vi "VPA QC Flow Calibration.vi"(9 "DAQ Ref Cluster":T2, 10 "State In":T4) -> (2 "State Out":T4)   [LabVIEW 2013]
uses:
  Controls/VPA QC State Data Cluster.ctl
  Controls/VPA QC General Cluster.ctl
  Controls/VPA QC State Enum.ctl
  Controls/VPA QC Bool Cluster.ctl
  Controls/VPA QC DAQ Ref Cluster.ctl
  Controls/VPA QC Scale Communication Settings DVR.ctl
  Controls/VPA QC Scale Communication Settings.ctl
  Controls/VPA QC Flow Rate Data Cluster.ctl
  Controls/VPA QC Volume Timer Enum.ctl
panel:
  in  "Flow Data Array":T1[](array[typedef])
  in  "Set 4":bool
  in  "Set 3":bool
  in  "Set 2":bool
  in  "Set 1":bool
  in  "Density of Fluid":dbl=0.996
  out "Cust 2 Elapsed Time":dbl format="%<%M:%S%1u>t"
  in  "Cust Rate 2":dbl=0.01 caption="ML/Min"
  in  "Cust Rate 1":dbl=0.1 caption="ML/Min"
  out "% Dif 4":dbl
  out "Volume 4":dbl caption="Flow Rate (mL/min)" format="%5.2g"
  out "Running 4":bool
  in  "Cust Ready 2":bool caption="Custom Timer2"
  out "Rate 4":dbl
  in  "Flow Rate 4":dbl caption="Flow Rate (mL/min)"
  out "Calc Vol 4":dbl
  out "% Difference Cust1":dbl
  out "Volume 3":dbl caption="Flow Rate (mL/min)" format="%5.2g"
  out "Running 3":bool
  in  "Cust Ready 1":bool caption="Custom Timer1"
  out "Cust 1 Calculated \nFlow Rate (mL/min)":dbl
  out "Cust 1 Elapsed Time":dbl format="%<%M:%S%1u>t"
  in  "Flow Rate 3":dbl caption="Flow Rate (mL/min)"
  out "Vol 3":dbl
  out "A Side Calibration Constant":dbl caption="Flow Rate (mL/min)"
  out "B Side Calibration Constant":dbl caption="Flow Rate (mL/min)"
  out "% Difference 100":dbl
  out "% Difference 50":dbl caption="% Difference"
  out "Volume 2":dbl caption="Flow Rate (mL/min)" format="%5.2g"
  out "Reported\nVolume":dbl caption="Flow Rate (mL/min)" format="%5.2g"
  in  "Cancel":bool
  in  "Save":bool
  out "Running 2":bool
  out "Running":bool
  in  "Ready 100%":bool caption="95% Flow Rate"
  in  "Ready 50%":bool caption="50% Flow Rate"
  out "Calculated Flow Rate\n(mL/min) 2":dbl
  out "Calculated Flow\n Rate (mL/min)":dbl
  out "Elapsed Time 2":dbl format="%<%M:%S%1u>t"
  out "Elapsed Time":dbl format="%<%M:%S%1u>t"
  in  "Flow Rate 2":dbl caption="Flow Rate (mL/min)"
  in  "Flow Rate\n(mL/min)":dbl caption="Flow Rate (mL/min)"
  out "Vol 2":dbl
  out "Vol 1":dbl caption="Measured\nVolume\n(mass/density)"
  # "Flow Rate Test"
  # "1. Go to Constant Flow Mode and flow to some volume at 50%  max flow, 95% max flow, and two low flow rates. Calculate the flow rate from the measured volume and time."
  # "Enter Pump\nReported Values"
  # "Calculated Values"
  # "Assembly Checklist"
  # "Assembly Checklist"
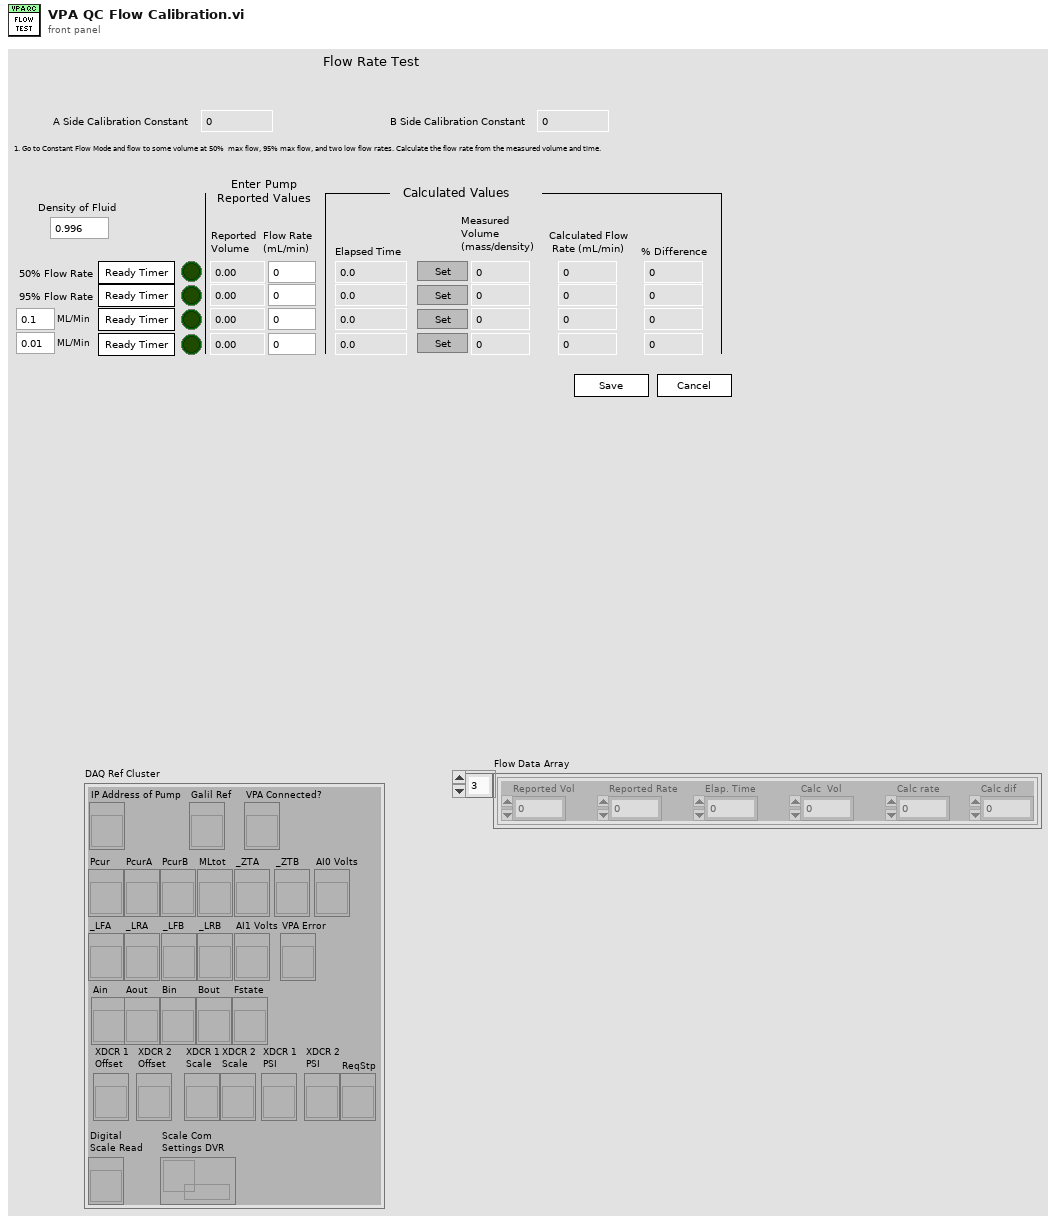
[diagram p1: front panel]
types:
  T1 = typedef "VPA QC Flow Rate Data Cluster.ctl" = cluster{"Reported Vol":dbl, "Reported Rate":dbl, "Elap. Time":dbl, "Calc  Vol":dbl, "Calc rate":dbl, "Calc dif":dbl}
  T2 = typedef "VPA QC DAQ Ref Cluster.ctl" = cluster{"IP Address of Pump":refnum<vi>, "Galil Ref":refnum<vi>, "VPA Connected?":refnum<vi>, "Pcur":refnum<vi>, "PcurA":refnum<vi>, "PcurB":refnum<vi>, "MLtot":refnum<vi>, "_LFA":refnum<vi>, "_LRA":refnum<vi>, "_LFB":refnum<vi>, "_LRB":refnum<vi>, "_ZTA":refnum<vi>, "_ZTB":refnum<vi>, "AI0 Volts":refnum<vi>, "AI1 Volts":refnum<vi>, "VPA Error":refnum<vi>, "Ain":refnum<vi>, "Aout":refnum<vi>, "Bin":refnum<vi>, "Bout":refnum<vi>, "Fstate":refnum<vi>, "XDCR 1\nOffset":refnum<vi>, "XDCR 2 \nOffset":refnum<vi>, "XDCR 1\nScale":refnum<vi>, "XDCR 2\nScale":refnum<vi>, "XDCR 1\nPSI":refnum<vi>, "XDCR 2\nPSI":refnum<vi>, "ReqStp":refnum<vi>, "Digital \nScale Read":refnum<vi>, "Scale Com\nSettings DVR":T3}
  T3 = typedef "VPA QC Scale Communication Settings DVR.ctl" = refnum<data-value>
  T4 = typedef "VPA QC State Data Cluster.ctl" = cluster{"XDCR 1":tag, "XDCR 2":tag, "General Information Clust":T5, "Assembly Checklist":cluster{"Ensure Drive Assembly checklist is completed.":bool, "Tighten Screws":bool, "Ensure VPA is wired correctly.":bool, "Ensure pump is running at voltage specified by customer.":bool}, "State":T6, "Manifold Leak Test Data":dbl[][], "Pressure Verification Test Data":dbl[][], "Flow Mode Verification Data":dbl[][], "DAQmx Error":errorcluster, "Bool Cluster":T7, "Leak Test Start Time":timestamp, "Pressure Test Start Time":timestamp, "Flow Test Start Time":timestamp, "Final Checklist cluster":cluster{"Check Fact Rest":bool, "Initialize Pump":bool, "Maintenance Hours":bool, "Clean Water Out":bool, "Covers":bool, "Screws":bool, "Wrap":bool, "Box":bool}, "Volts Constant":dbl, "Volume Constant A":dbl, "Volume Constant B":dbl, "Save File Path":path, "Comments Array":string[][], "File Format Version":u16}
  T5 = typedef "VPA QC General Cluster.ctl" = cluster{"Tech Name":string, "Date":timestamp, "Customer":string, "VPA Model":string, "G-72 Software Version":string, "Galil SN":string, "Galil Software Version":string, "VPA SN":string, "Valve SN":string, "Side A Drive Module SN":string, "Side B Drive Module SN":string, "A Side Transducer SN":string, "B Side Transducer SN":string, "A Side Motor SN":string, "B Side Motor SN":string, "A Side Gear Reducer SN":string, "B Side Gear Reducer SN":string, "A Side Limit Switch SN":string, "B Side Limit Switch SN":string, "Pump Voltage":string}
  T6 = typedef "VPA QC State Enum.ctl" = enum16{"General Information", "XDCR and LS Check", "Check Pump Function", "Manifold/Cylinder Leak Test", "Exit"}
  T7 = typedef "VPA QC Bool Cluster.ctl" = cluster{"Assembly":bool, "Gen":bool, "XDCR and LS Setup":bool, "Verify Pump Operation":bool, "Leak Test":bool, "Calibrate XDCRs":bool, "P Mode Verify":bool, "F Mode Verify":bool, "Vol Calibration":bool, "Flow Rate Test":bool, "Final Checklist":bool}
  T8 = enum8{"Enabled", "Disabled", "Disabled and Grayed Out"}
  T9 = typedef "VPA QC Volume Timer Enum.ctl" = enum16{"Idle", "50% Watch Ready", "100% Watch Ready", "50% Timer Running", "100% Timer Running", "Cust1 Timer Ready", "Cust1 Timer Running", "Cust2 Timer Ready", "Cust2 Timer Running"}
  T10 = cluster{"Reported Vol":dbl, "Reported Rate":dbl, "Elap. Time":dbl, "Calc  Vol":dbl, "Calc rate":dbl, "Calc dif":dbl}[]
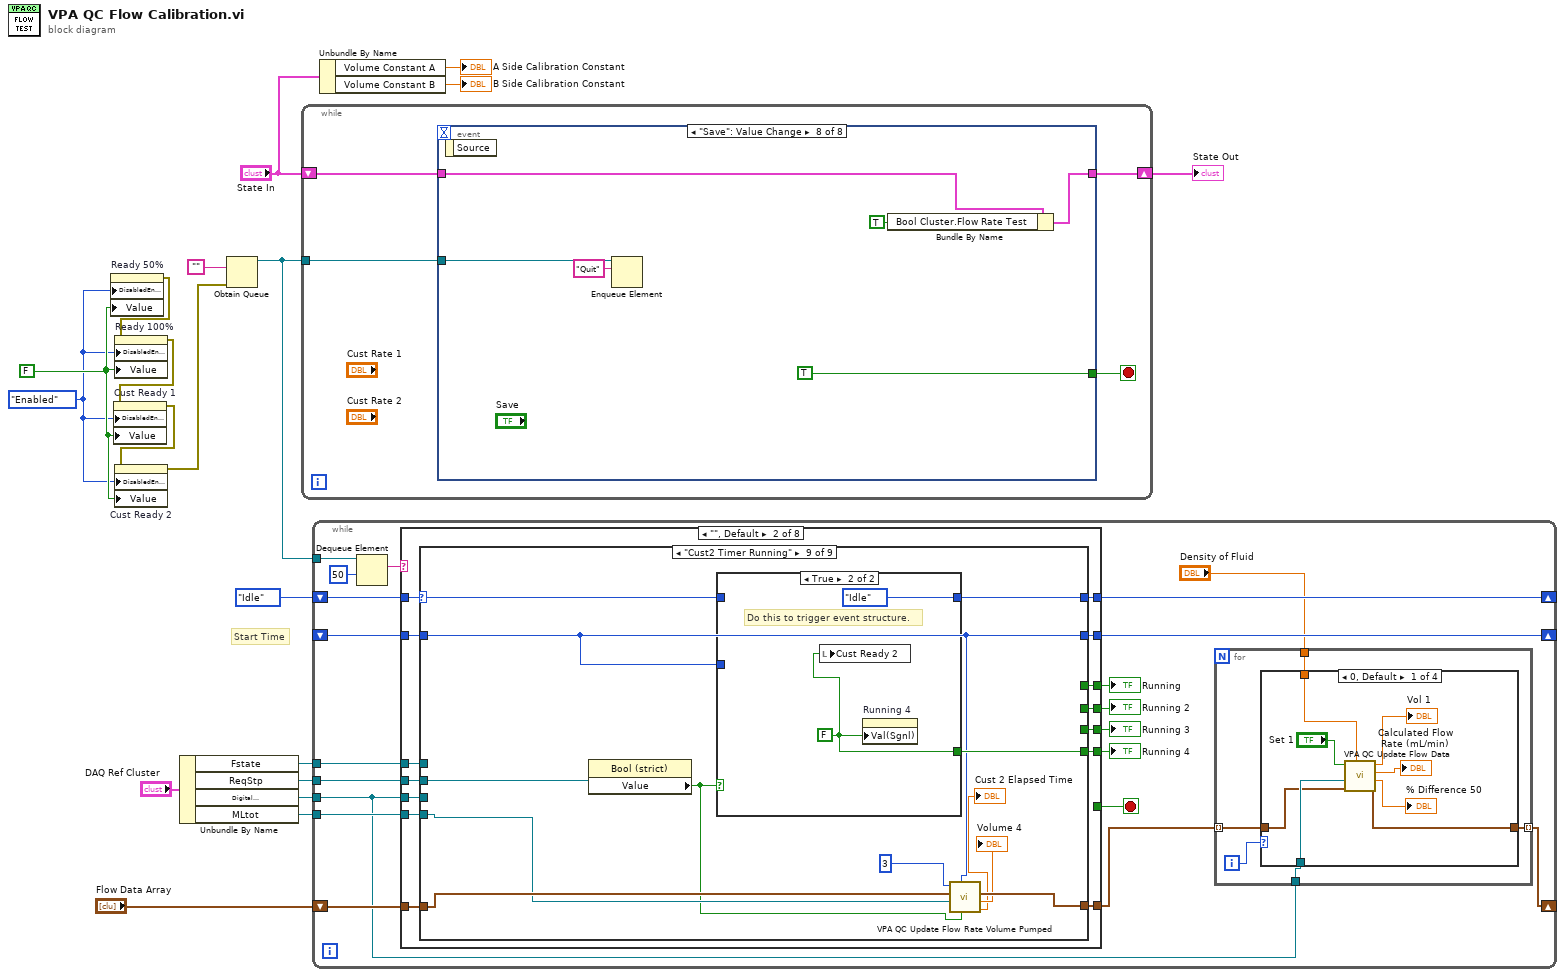
[diagram p0: block diagram]
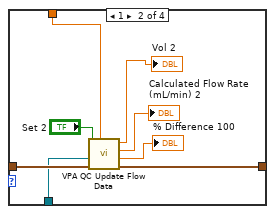
[diagram p2: hidden frame]
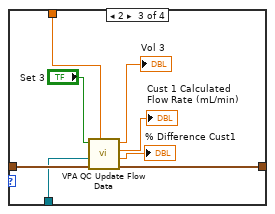
[diagram p3: hidden frame]
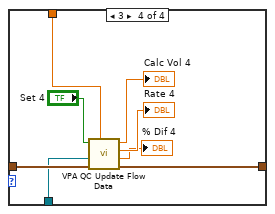
[diagram p4: hidden frame]
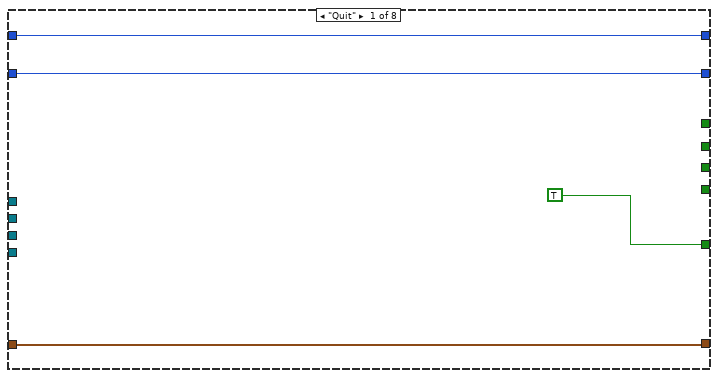
[diagram p5: hidden frame]
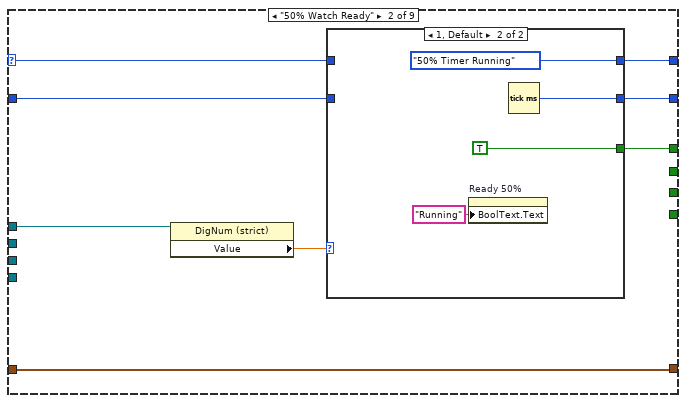
[diagram p7: hidden frame]
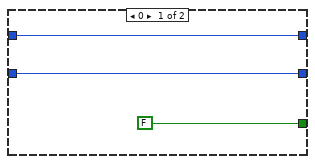
[diagram p8: hidden frame]
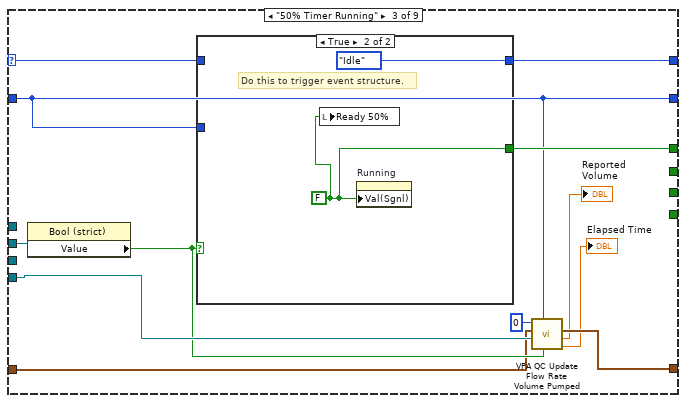
[diagram p9: hidden frame]
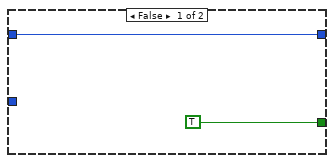
[diagram p10: hidden frame]
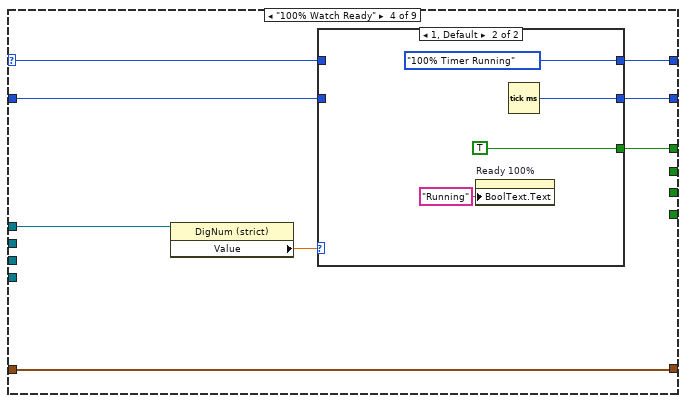
[diagram p11: hidden frame]
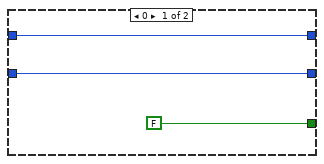
[diagram p12: hidden frame]
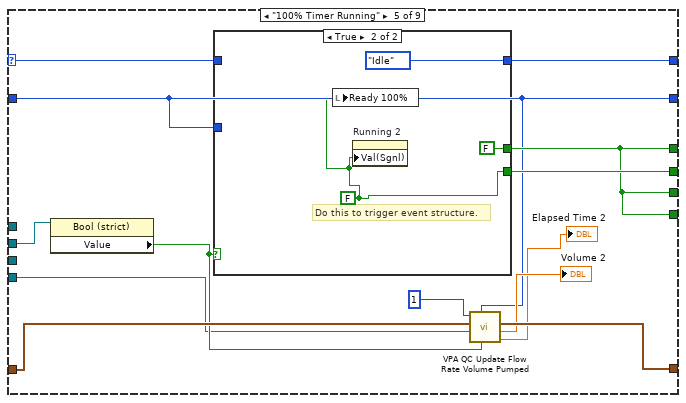
[diagram p13: hidden frame]
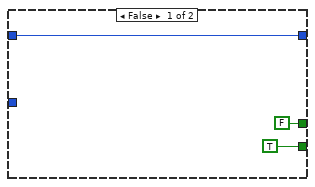
[diagram p14: hidden frame]
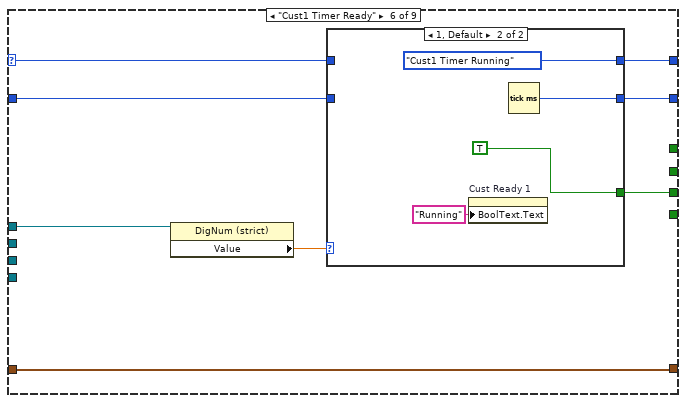
[diagram p15: hidden frame]
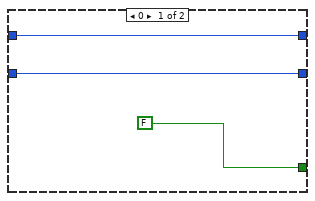
[diagram p16: hidden frame]
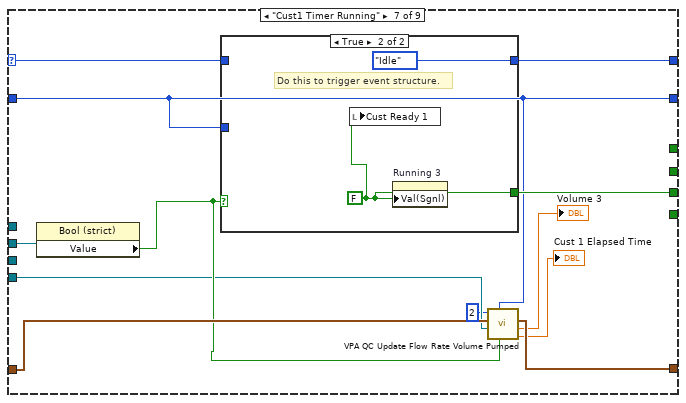
[diagram p17: hidden frame]
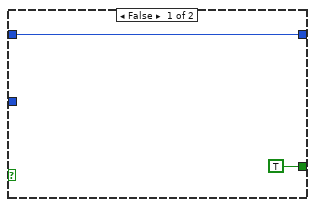
[diagram p18: hidden frame]
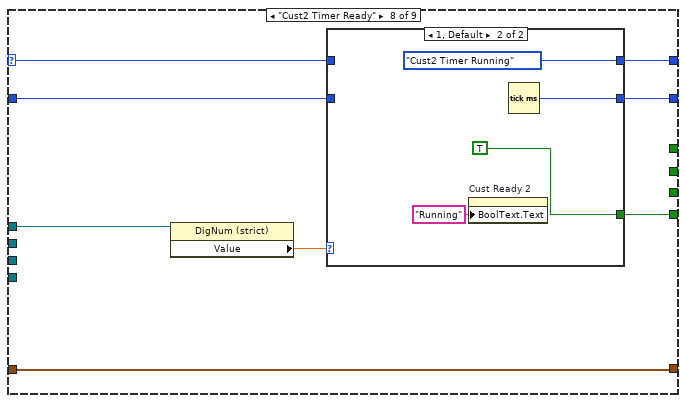
[diagram p19: hidden frame]
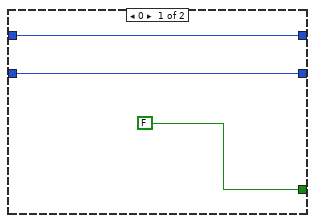
[diagram p20: hidden frame]
diagram:
  w6 = FALSE ("Ready 50%")
  w5 = T8."Enabled" ("Disabled")
  # "Start Time"
  n1 = property on="Ready 50%" class="Bool (strict)"("DisabledEnum"=w5, "Value"=w6) -> (error out=w4:errorcluster)  [unwired: 2 in, 1 out]
  n2 = property on="Ready 100%" class="Bool (strict)"(error in=w4, "DisabledEnum"=w5, "Value"=w6) -> (error out=w3:errorcluster)  [unwired: 1 in, 1 out]
  n3 = property on="Cust Ready 1" class="Bool (strict)"(error in=w3, "DisabledEnum"=w5, "Value"=w6) -> (error out=w2:errorcluster)  [unwired: 1 in, 1 out]
  n4 = property on="Cust Ready 2" class="Bool (strict)"(error in=w2, "DisabledEnum"=w5, "Value"=w6) -> (error out=w1:errorcluster)  [unwired: 1 in, 1 out]
  n5 = Unbundle By Name("DAQ Ref Cluster") -> ("Fstate"=w15:refnum<vi>, "ReqStp"=w13:refnum<vi>, "Digital \nScale Read"=w11:refnum<vi>, "MLtot"=w8:refnum<vi>)
  n6 = Obtain Queue(element data type="", error in (no error)=w1) -> (queue out=w17:refnum<queue>)  [unwired: 3 in, 2 out]
  n7 = while {
    shift-right: [w21] -> w19
    shift-left: "State In" -> [w22]
    tunnel: w17 -> [w20]
    stop <- w23 stop-if-true
    n8 = event shown="[7] \"Save\": Value Change" {
      selector: _ -> [_ _ _ _ _ _ _ _]
      dyn-events: _ -> [_ _ _ _ _ _ _ _]
      timeout: _ -> [_ _ _ _ _ _ _ _]
      tunnel: [TRUE _ _ _ _ _ _ TRUE] -> w23
      tunnel: w22 -> [w26 w33 w45 w57 w69 w78 w81 w86]
      tunnel: [w26 w33 w45 w57 w69 w78 w81 w85] -> w21
      tunnel: w20 -> [w25 w32 w44 w56 w68 w77 _ w83]
      event "Cancel": Value Change {
        n9 = event-data() -> ()  [unwired: 1 in, 1 out]
        n10 = Enqueue Element(queue=w25, element="Quit") -> ()  [unwired: 2 in, 3 out]
      }
      event "Ready 50%": Value Change {
        n11 = event-data() -> ()  [unwired: 1 in, 1 out]
        n12 = case shown="False" "Ready 50%" {
          tunnel: ["Cancel Timer" ("element") "Start 50% Watch" ("element")] -> w31
          tunnel: ["Ready Timer" ("Boolean Text.Text") "Waiting..." ("Boolean Text.Text")] -> w30
          tunnel: [0 2] -> w28
          frame False {
          }
          frame True {
          }
        }
        n13 = Enqueue Element(queue=w32, element=w31) -> ()  [unwired: 2 in, 3 out]
        n14 = property on="Ready 50%" class="Bool (strict)"("BoolText.Text"=w30) -> ()  [unwired: 2 in, 2 out]
        n15 = property on="Ready 100%" class="Bool (strict)"("DisabledEnum"=w28) -> ()  [unwired: 2 in, 2 out]
        n16 = property on="Cust Ready 1" class="Bool (strict)"("DisabledEnum"=w28) -> ()  [unwired: 2 in, 2 out]
        n17 = property on="Cust Ready 2" class="Bool (strict)"("DisabledEnum"=w28) -> ()  [unwired: 2 in, 2 out]
      }
      event "Ready 100%": Value Change {
        n18 = event-data() -> ()  [unwired: 1 in, 1 out]
        n19 = case shown="True" "Ready 100%" {
          tunnel: ["Cancel Timer" ("element") "Start 100% Watch" ("element")] -> w43
          tunnel: ["Ready Timer" ("Boolean Text.Text") "Waiting..." ("Boolean Text.Text")] -> w42
          tunnel: [0 2] -> w40
          frame False {
          }
          frame True {
          }
        }
        n20 = property on="Ready 100%" class="Bool (strict)"("BoolText.Text"=w42) -> ()  [unwired: 2 in, 2 out]
        n21 = Enqueue Element(queue=w44, element=w43) -> ()  [unwired: 2 in, 3 out]
        n22 = property on="Ready 50%" class="Bool (strict)"("DisabledEnum"=w40) -> ()  [unwired: 2 in, 2 out]
        n23 = property on="Cust Ready 1" class="Bool (strict)"("DisabledEnum"=w40) -> ()  [unwired: 2 in, 2 out]
        n24 = property on="Cust Ready 2" class="Bool (strict)"("DisabledEnum"=w40) -> ()  [unwired: 2 in, 2 out]
      }
      event "Cust Ready 1": Value Change {
        n25 = event-data() -> ()  [unwired: 1 in, 1 out]
        n26 = case shown="False" "Cust Ready 1" {
          tunnel: ["Cancel Timer" ("element") "Start Cust Timer 1" ("element")] -> w55
          tunnel: ["Ready Timer" ("Boolean Text.Text") "Waiting..." ("Boolean Text.Text")] -> w54
          tunnel: [0 2] -> w52
          frame False {
          }
          frame True {
          }
        }
        n27 = property on="Cust Ready 1" class="Bool (strict)"("BoolText.Text"=w54) -> ()  [unwired: 2 in, 2 out]
        n28 = Enqueue Element(queue=w56, element=w55) -> ()  [unwired: 2 in, 3 out]
        n29 = property on="Ready 50%" class="Bool (strict)"("DisabledEnum"=w52) -> ()  [unwired: 2 in, 2 out]
        n30 = property on="Ready 100%" class="Bool (strict)"("DisabledEnum"=w52) -> ()  [unwired: 2 in, 2 out]
        n31 = property on="Cust Ready 2" class="Bool (strict)"("DisabledEnum"=w52) -> ()  [unwired: 2 in, 2 out]
      }
      event "Cust Ready 2": Value Change {
        n32 = event-data() -> ()  [unwired: 1 in, 1 out]
        n33 = case shown="False" "Cust Ready 2" {
          tunnel: ["Cancel Timer" ("element") "Start Cust Timer 2" ("element")] -> w67
          tunnel: ["Ready Timer" ("Boolean Text.Text") "Waiting..." ("Boolean Text.Text")] -> w66
          tunnel: [0 2] -> w64
          frame False {
          }
          frame True {
          }
        }
        n34 = property on="Cust Ready 2" class="Bool (strict)"("BoolText.Text"=w66) -> ()  [unwired: 2 in, 2 out]
        n35 = Enqueue Element(queue=w68, element=w67) -> ()  [unwired: 2 in, 3 out]
        n36 = property on="Ready 50%" class="Bool (strict)"("DisabledEnum"=w64) -> ()  [unwired: 2 in, 2 out]
        n37 = property on="Ready 100%" class="Bool (strict)"("DisabledEnum"=w64) -> ()  [unwired: 2 in, 2 out]
        n38 = property on="Cust Ready 1" class="Bool (strict)"("DisabledEnum"=w64) -> ()  [unwired: 2 in, 2 out]
      }
      event "Flow Rate\n(mL/min)", "Flow Rate 2", "Flow Rate 4", "Flow Rate 3": Value Change {
        n39 = event-data() -> ()  [unwired: 1 in, 6 out]
        n40 = Enqueue Element(queue=w77, element="Update Set Rate") -> ()  [unwired: 2 in, 3 out]
      }
      event "Running", "Running 2", "Running 3", "Running 4": Value Change {
        w79 = FALSE ("Ready 50%")
        w80 = T8."Enabled" ("Disabled")
        n41 = event-data() -> ()  [unwired: 1 in, 1 out]
        n42 = property on="Ready 50%" class="Bool (strict)"("DisabledEnum"=w80, "Value"=w79) -> ()  [unwired: 2 in, 2 out]
        n43 = property on="Cust Ready 1" class="Bool (strict)"("DisabledEnum"=w80, "Value"=w79) -> ()  [unwired: 2 in, 2 out]
        n44 = property on="Ready 100%" class="Bool (strict)"("DisabledEnum"=w80, "Value"=w79) -> ()  [unwired: 2 in, 2 out]
        n45 = property on="Cust Ready 2" class="Bool (strict)"("DisabledEnum"=w80, "Value"=w79) -> ()  [unwired: 2 in, 2 out]
      }
      event "Save": Value Change {
        n46 = event-data() -> ()  [unwired: 1 in, 1 out]
        n47 = Enqueue Element(queue=w83, element="Quit") -> ()  [unwired: 2 in, 3 out]
        n48 = Bundle By Name(cluster=w86, "Bool Cluster.Flow Rate Test"=TRUE ("Bool Cluster.Vol Calibration")) -> (w85:T4)
      }
    }
  }
  "State Out" <- w19
  n49 = while {
    tunnel: w17 -> [w107]
    shift-right: [w100] -> _
    shift-left: VPA_QC_Volume_Timer_Enum."Idle" ("Enum") -> [w99]
    shift-right: [w103] -> _
    shift-left: _ -> [w102]
    tunnel: w15 -> [w101]
    tunnel: w13 -> [w96]
    tunnel: w11 -> [w90]
    tunnel: w8 -> [w93]
    shift-right: [w88] -> _
    shift-left: "Flow Data Array" -> [w92]
    stop <- w105 stop-if-true
    n50 = Dequeue Element(queue=w107, timeout in ms (-1)=50) -> (element=w106:string)  [unwired: 1 in, 3 out]
    n51 = case shown="\"\", Default" w106 {
      tunnel: [TRUE _ _ _ _ _ _ _] -> w105
      tunnel: [w147 w160 VPA_QC_Volume_Timer_Enum."50% Watch Ready" ("Enum") VPA_QC_Volume_Timer_Enum."100% Watch Ready" ("Enum") VPA_QC_Volume_Timer_Enum."Cust1 Timer Ready" ("Enum") VPA_QC_Volume_Timer_Enum."Cust2 Timer Ready" ("Enum") VPA_QC_Volume_Timer_Enum."Idle" ("Enum") w311] -> w100
      tunnel: w99 -> [w147 w162 _ _ _ _ _ w311]
      tunnel: [w146 w157 w295 w297 w300 w303 w307 w310] -> w103
      tunnel: w102 -> [w146 w158 w295 w297 w300 w303 w307 w310]
      tunnel: w101 -> [_ w161 _ _ _ _ _ _]
      tunnel: [_ w159 _ _ _ _ _ _] -> w98
      tunnel: [_ w156 _ _ _ _ _ _] -> w97
      tunnel: w96 -> [_ w155 _ _ _ _ _ _]
      tunnel: [_ w154 _ _ _ _ _ _] -> w95
      tunnel: [_ w153 _ _ _ _ _ _] -> w94
      tunnel: w90 -> [_ w152 _ _ _ _ _ _]
      tunnel: w93 -> [_ w151 _ _ _ _ _ _]
      tunnel: w92 -> [w145 w150 w293 w296 w299 w302 w305 w309]
      tunnel: [w145 w149 w293 w296 w299 w302 w305 w308] -> w89
      frame "Quit" {
      }
      frame "", Default {
        n52 = case shown="\"Cust2 Timer Running\"" w162 {
          selector: w162 -> [w165 w171 w191 w202 w223 w236 w256 w267 w287]
          tunnel: w161 -> [_ w173 _ w204 _ w238 _ w269 _]
          tunnel: w158 -> [w164 w167 w186 w198 w213 w233 w246 w264 w281]
          tunnel: [w165 w170 w192 w201 w224 w235 w257 w266 w288] -> w160
          tunnel: [_ w169 w190 w200 w220 _ _ _ _] -> w159
          tunnel: [w164 w168 w186 w199 w213 w234 w246 w265 w281] -> w157
          tunnel: [_ _ _ _ w222 _ _ _ _] -> w156
          tunnel: w155 -> [_ _ w189 _ w221 _ w255 _ w286]
          tunnel: [_ _ _ _ w220 w232 w254 _ _] -> w154
          tunnel: [_ _ _ _ w220 _ _ w263 w285] -> w153
          tunnel: w152 -> [_ _ _ _ _ _ _ _ _]
          tunnel: w151 -> [_ _ w188 _ w212 _ w248 _ w280]
          tunnel: w150 -> [w163 w166 w184 w197 w219 w231 w253 w262 w284]
          tunnel: [w163 w166 w183 w197 w218 w231 w252 w262 w283] -> w149
          frame "Idle" {
          }
          frame "50% Watch Ready" {
            n53 = property class="DigNum (strict)"(reference=w173) -> ("Value"=w172:dbl)  [unwired: 1 in, 2 out]
            n54 = case shown="1, Default" w172 {
              tunnel: w171 -> [w175 _]
              tunnel: [w175 VPA_QC_Volume_Timer_Enum."50% Timer Running" ("Enum")] -> w170
              tunnel: [FALSE TRUE] -> w169
              tunnel: [w174 w178] -> w168
              tunnel: w167 -> [w174 _]
              frame 0 {
              }
              frame 1, Default {
                n55 = property on="Ready 50%" class="Bool (strict)"("BoolText.Text"="Running" ("Boolean Text.Text")) -> ()  [unwired: 2 in, 2 out]
                n56 = Tick Count (ms)() -> (millisecond timer value=w178:u32)
              }
            }
          }
          frame "50% Timer Running" {
            n57 = property class="Bool (strict)"(reference=w189) -> ("Value"=w187:bool)  [unwired: 1 in, 2 out]
            n58 = case shown="True" w187 {
              tunnel: w186 -> [_ _]
              tunnel: [w194 VPA_QC_Volume_Timer_Enum."Idle" ("Enum")] -> w192
              tunnel: w191 -> [w194 _]
              tunnel: [TRUE w195] -> w190
              frame False {
              }
              frame True {
                w195 = FALSE
                # "Do this to trigger event structure."
                n59 = local write "Ready 50%"(w195) -> ()
                n60 = property on="Running" class="Bool (strict)"("Val(Sgnl)"=w195) -> ()  [unwired: 2 in, 2 out]
              }
            }
            n61 = call "VPA QC Update Flow Rate Volume Pumped.vi"("ReqStp?"=w187, "MS Time"=w186, "MLtot"=w188, "Flow Rate Data In"=w184, "Test #"=i8 0) -> ("Elapsed Time"=→"Elapsed Time":dbl, "Volume"=→"Reported\nVolume":dbl, "Flow Data Out"=w183:T10)  [unwired: 4 in]
          }
          frame "100% Watch Ready" {
            n62 = property class="DigNum (strict)"(reference=w204) -> ("Value"=w203:dbl)  [unwired: 1 in, 2 out]
            n63 = case shown="1, Default" w203 {
              tunnel: w202 -> [w206 _]
              tunnel: [w206 VPA_QC_Volume_Timer_Enum."100% Timer Running" ("Enum")] -> w201
              tunnel: [FALSE TRUE] -> w200
              tunnel: [w205 w209] -> w199
              tunnel: w198 -> [w205 _]
              frame 0 {
              }
              frame 1, Default {
                n64 = property on="Ready 100%" class="Bool (strict)"("BoolText.Text"="Running" ("Boolean Text.Text")) -> ()  [unwired: 2 in, 2 out]
                n65 = Tick Count (ms)() -> (millisecond timer value=w209:u32)
              }
            }
          }
          frame "100% Timer Running" {
            n66 = property class="Bool (strict)"(reference=w221) -> ("Value"=w215:bool)  [unwired: 1 in, 2 out]
            n67 = case shown="True" w215 {
              tunnel: w213 -> [_ _]
              tunnel: [w227 VPA_QC_Volume_Timer_Enum."Idle" ("Enum")] -> w224
              tunnel: w223 -> [w227 _]
              tunnel: [FALSE FALSE] -> w220
              tunnel: [TRUE w228] -> w222
              frame False {
              }
              frame True {
                w228 = FALSE
                # "Do this to trigger event structure."
                n68 = local write "Ready 100%"(w228) -> ()
                n69 = property on="Running 2" class="Bool (strict)"("Val(Sgnl)"=w228) -> ()  [unwired: 2 in, 2 out]
              }
            }
            n70 = call "VPA QC Update Flow Rate Volume Pumped.vi"("ReqStp?"=w215, "MS Time"=w213, "MLtot"=w212, "Flow Rate Data In"=w219, "Test #"=1 ("index")) -> ("Elapsed Time"=→"Elapsed Time 2":dbl, "Volume"=→"Volume 2":dbl, "Flow Data Out"=w218:T10)  [unwired: 4 in]
          }
          frame "Cust1 Timer Ready" {
            n71 = property class="DigNum (strict)"(reference=w238) -> ("Value"=w237:dbl)  [unwired: 1 in, 2 out]
            n72 = case shown="1, Default" w237 {
              tunnel: w236 -> [w240 _]
              tunnel: [w240 VPA_QC_Volume_Timer_Enum."Cust1 Timer Running" ("Enum")] -> w235
              tunnel: [FALSE TRUE] -> w232
              tunnel: [w239 w243] -> w234
              tunnel: w233 -> [w239 _]
              frame 0 {
              }
              frame 1, Default {
                n73 = property on="Cust Ready 1" class="Bool (strict)"("BoolText.Text"="Running" ("Boolean Text.Text")) -> ()  [unwired: 2 in, 2 out]
                n74 = Tick Count (ms)() -> (millisecond timer value=w243:u32)
              }
            }
          }
          frame "Cust1 Timer Running" {
            n75 = property class="Bool (strict)"(reference=w255) -> ("Value"=w249:bool)  [unwired: 1 in, 2 out]
            n76 = case shown="True" w249 {
              tunnel: w246 -> [_ _]
              tunnel: [w259 VPA_QC_Volume_Timer_Enum."Idle" ("Enum")] -> w257
              tunnel: w256 -> [w259 _]
              tunnel: [TRUE w260] -> w254
              frame False {
              }
              frame True {
                w260 = FALSE
                # "Do this to trigger event structure."
                n77 = local write "Cust Ready 1"(w260) -> ()
                n78 = property on="Running 3" class="Bool (strict)"("Val(Sgnl)"=w260) -> ()  [unwired: 2 in, 2 out]
              }
            }
            n79 = call "VPA QC Update Flow Rate Volume Pumped.vi"("ReqStp?"=w249, "MS Time"=w246, "MLtot"=w248, "Flow Rate Data In"=w253, "Test #"=i8 2) -> ("Elapsed Time"=→"Cust 1 Elapsed Time":dbl, "Volume"=→"Volume 3":dbl, "Flow Data Out"=w252:T10)  [unwired: 4 in]
          }
          frame "Cust2 Timer Ready" {
            n80 = property class="DigNum (strict)"(reference=w269) -> ("Value"=w268:dbl)  [unwired: 1 in, 2 out]
            n81 = case shown="1, Default" w268 {
              tunnel: w267 -> [w271 _]
              tunnel: [w271 VPA_QC_Volume_Timer_Enum."Cust2 Timer Running" ("Enum")] -> w266
              tunnel: [FALSE TRUE] -> w263
              tunnel: [w270 w274] -> w265
              tunnel: w264 -> [w270 _]
              frame 0 {
              }
              frame 1, Default {
                n82 = property on="Cust Ready 2" class="Bool (strict)"("BoolText.Text"="Running" ("Boolean Text.Text")) -> ()  [unwired: 2 in, 2 out]
                n83 = Tick Count (ms)() -> (millisecond timer value=w274:u32)
              }
            }
          }
          frame "Cust2 Timer Running" {
            n84 = property class="Bool (strict)"(reference=w286) -> ("Value"=w279:bool)  [unwired: 1 in, 2 out]
            n85 = case shown="True" w279 {
              tunnel: w281 -> [_ _]
              tunnel: [w290 VPA_QC_Volume_Timer_Enum."Idle" ("Enum")] -> w288
              tunnel: w287 -> [w290 _]
              tunnel: [TRUE w291] -> w285
              frame False {
              }
              frame True {
                w291 = FALSE
                # "Do this to trigger event structure."
                n86 = local write "Cust Ready 2"(w291) -> ()
                n87 = property on="Running 4" class="Bool (strict)"("Val(Sgnl)"=w291) -> ()  [unwired: 2 in, 2 out]
              }
            }
            n88 = call "VPA QC Update Flow Rate Volume Pumped.vi"("ReqStp?"=w279, "MS Time"=w281, "MLtot"=w280, "Flow Rate Data In"=w284, "Test #"=3 ("index")) -> ("Elapsed Time"=→"Cust 2 Elapsed Time":dbl, "Volume"=→"Volume 4":dbl, "Flow Data Out"=w283:T10)  [unwired: 4 in]
          }
        }
      }
      frame "Start 50% Watch" {
      }
      frame "Start 100% Watch" {
      }
      frame "Start Cust Timer 1" {
      }
      frame "Start Cust Timer 2" {
      }
      frame "Cancel Timer" {
      }
      frame "Update Set Rate" {
        n89 = for {
          tunnel: w309 -> [w314] mode=indexing
          tunnel: [w312] -> w308 mode=indexing
          i -> [w313]
          n90 = case shown="3" w313 {
            tunnel: w314 -> [w317 w320 w323 w326]
            tunnel: [w315 w319 w322 w325] -> w312
            frame 0, Default {
              n91 = Bundle By Name(cluster=w317, "Reported Rate"="Flow Rate\n(mL/min)") -> (w315:T1)
            }
            frame 1 {
              n92 = Bundle By Name(cluster=w320, "Reported Rate"="Flow Rate 2") -> (w319:T1)
            }
            frame 2 {
              n93 = Bundle By Name(cluster=w323, "Reported Rate"="Flow Rate 3") -> (w322:T1)
            }
            frame 3 {
              n94 = Bundle By Name(cluster=w326, "Reported Rate"="Flow Rate 4") -> (w325:T1)
            }
          }
        }
      }
    }
    "Running" <- w98
    "Running 2" <- w97
    "Running 3" <- w95
    "Running 4" <- w94
    n95 = for {
      tunnel: w89 -> [w111] mode=indexing
      tunnel: "Density of Fluid" -> [w110]
      tunnel: w90 -> [w109]
      tunnel: [w108] -> w88 mode=indexing
      i -> [w112]
      n96 = case shown="0, Default" w112 {
        tunnel: w111 -> [w117 w128 w136 w144]
        tunnel: w110 -> [w119 w126 w133 w139]
        tunnel: w109 -> [w118 w124 w132 w141]
        tunnel: [w113 w127 w135 w143] -> w108
        frame 0, Default {
          n97 = call "VPA QC Update Flow Data.vi"("Density of Fluid"=w119, "Flow Rate Test Data"=w117, "Digital \nScale Read"=w118, "Set"="Set 1") -> ("Rate Data Out"=w113:T1, "% Difference"=→"% Difference 50":dbl, "Flow Rate"=→"Calculated Flow\n Rate (mL/min)":dbl, "Calculated Volume"=→"Vol 1":dbl)  [unwired: 4 in]
        }
        frame 1 {
          n98 = call "VPA QC Update Flow Data.vi"("Density of Fluid"=w126, "Flow Rate Test Data"=w128, "Digital \nScale Read"=w124, "Set"="Set 2") -> ("Rate Data Out"=w127:T1, "% Difference"=→"% Difference 100":dbl, "Flow Rate"=→"Calculated Flow Rate\n(mL/min) 2":dbl, "Calculated Volume"=→"Vol 2":dbl)  [unwired: 4 in]
        }
        frame 2 {
          n99 = call "VPA QC Update Flow Data.vi"("Density of Fluid"=w133, "Flow Rate Test Data"=w136, "Digital \nScale Read"=w132, "Set"="Set 3") -> ("Rate Data Out"=w135:T1, "% Difference"=→"% Difference Cust1":dbl, "Flow Rate"=→"Cust 1 Calculated \nFlow Rate (mL/min)":dbl, "Calculated Volume"=→"Vol 3":dbl)  [unwired: 4 in]
        }
        frame 3 {
          n100 = call "VPA QC Update Flow Data.vi"("Density of Fluid"=w139, "Flow Rate Test Data"=w144, "Digital \nScale Read"=w141, "Set"="Set 4") -> ("Rate Data Out"=w143:T1, "% Difference"=→"% Dif 4":dbl, "Flow Rate"=→"Rate 4":dbl, "Calculated Volume"=→"Calc Vol 4":dbl)  [unwired: 4 in]
        }
      }
    }
  }
  n101 = Unbundle By Name("State In") -> ("Volume Constant A"=→"A Side Calibration Constant":dbl, "Volume Constant B"=→"B Side Calibration Constant":dbl)
